vi "Test sound.vi"() -> ()   [LabVIEW 2019]
panel:
  in  "index":i32
  in  "stop":bool
  out "error out":errorcluster
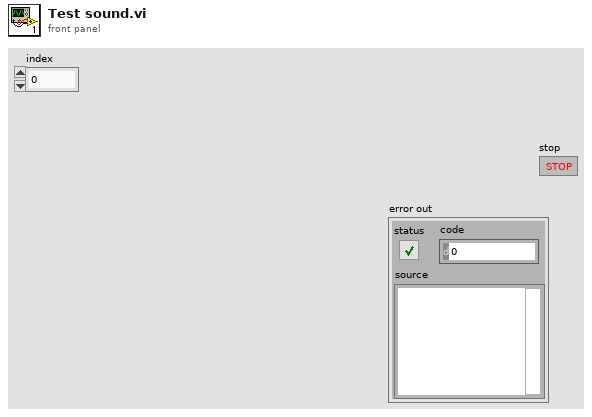
[diagram p1: front panel]
types:
  T1 = typedef "Sound Output Task ID.ctl" = u32
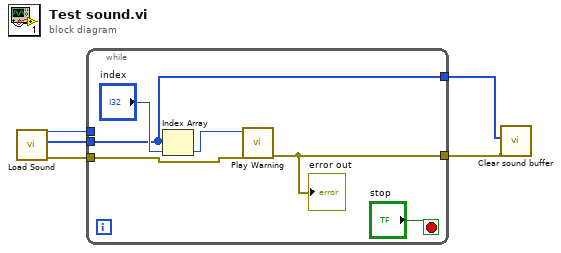
[diagram p0: block diagram]
diagram:
  n1 = call "Load Sound.vi"() -> ("error out"=w4:errorcluster, "Array"=w5:T1[], "task ID out"=w3:T1)  [unwired: 9 in]
  n2 = while {
    tunnel: w5 -> [w6]
    tunnel: w4 -> [w11]
    tunnel: w3 -> [_]
    tunnel: [w9] -> w2
    tunnel: [w6] -> w1
    stop <- "stop" stop-if-true
    n3 = Index Array(array=w6, index="index") -> (element=w8:T1)
    n4 = call "Play Warning.vi"("error in (no error)"=w11, "task ID"=w8) -> ("error out"=w9:errorcluster)  [unwired: 8 in, 1 out]
    "error out" <- w9
  }
  n5 = call "Clear sound buffer.vi"("error in (no error)"=w2, "array"=w1) -> ()  [unwired: 9 in, 1 out]
